vi "MathUtil_AngleModulus.vi"(11 "InputAngle":dbl) -> (3 "ModulsAngle":dbl)   [LabVIEW 2019, in "Trajectory_Library.lvlib"]
doc: "Wraps an angle to the range -pi to pi radians.\n \nInputs:\n - angleRadians -- Angle to wrap in radians.\n\nOutputs:\n - modulusAngle -- The wrapped angle."
uses:
  Trajectory_Library.lvlib
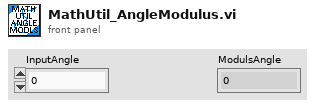
[diagram p1: front panel]
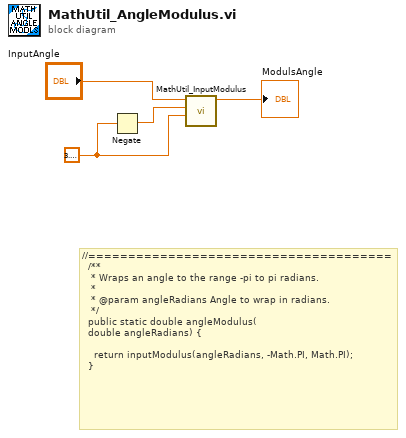
[diagram p0: block diagram]
diagram:
  w1 = 3.141592653589793
  # "//======================================\n  /**\n   * Wraps an angle to the range -pi to pi radians.\n   *\n   * @param angleRadians Angle to wrap in radians.\n   */\n  public static double angleModulus(\n\t\tdouble angleRadians) {\n\n    return inputModulus(angleRadians, -Math.PI, Math.PI);\n  }"
  n1 = Negate(x=w1) -> (-x=w2:dbl)
  n2 = call "MathUtil_InputModulus.vi"("Maximum_Input"=w1, "Minimum_Input"=w2, "Input"="InputAngle") -> ("modulus"=→"ModulsAngle":dbl)  [unwired: 8 in]
